vi "Module Top Level.vi"(8 "error in":errorcluster) -> (0 "error out":errorcluster)   [LabVIEW 2020, in "Error Handler.lvlib"]
doc: "This is the top level of the error handler module (a free running module of the ATM simulator). \n\nIt is closed using a user event or a local Stop button. It communicates with the other modules using a\nqueue based API which has comms modules that can be swapped if required."
uses:
  Error Handler.lvlib
  User Events/Controls/UE Abort Action.ctl
  Private Controls/Module Action.ctl
  Private Controls/Module Data Cluster.ctl
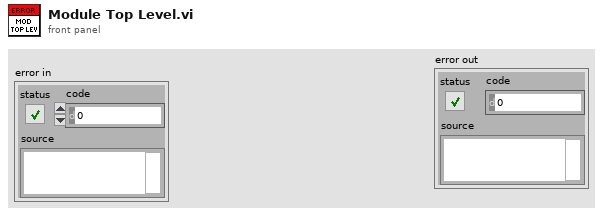
[diagram p1: front panel]
types:
  T1 = typedef "Error Handler.lvlib/Module Data Cluster.ctl" = cluster{"Data":variant, "Action":T2}
  T2 = typedef "Error Handler.lvlib/Module Action.ctl" = enum16{"Process_Step_Err", "Sensor_IO_err", "User_Console_err", "Display_Consol_err", "Error_Log", "Error", "Exit", "Init"}
  T3 = typedef "UE Abort Action.ctl" = enum16{"Destroy", "Get", "Create"}
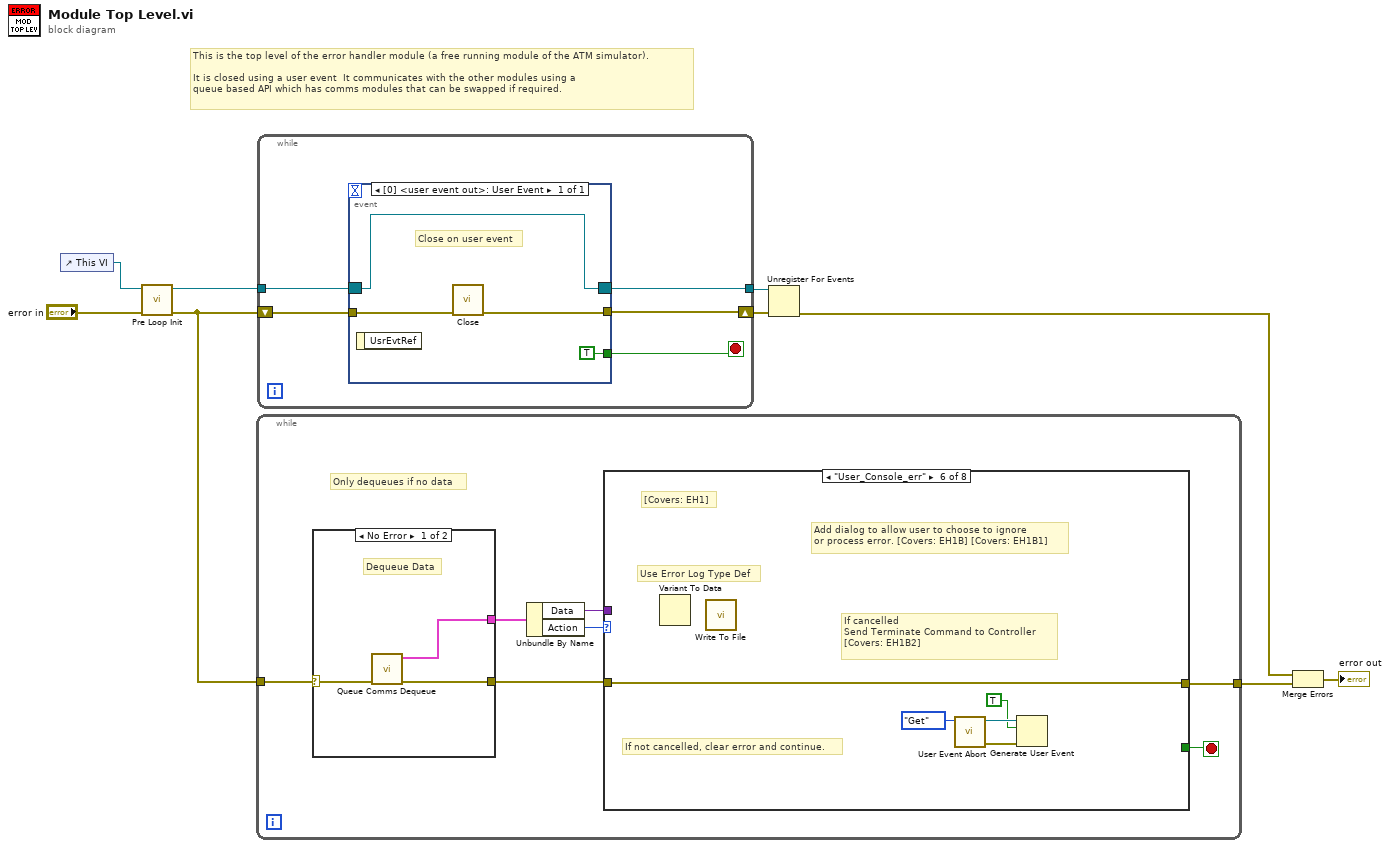
[diagram p0: block diagram]
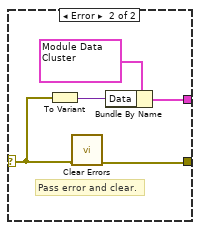
[diagram p2: hidden frame]
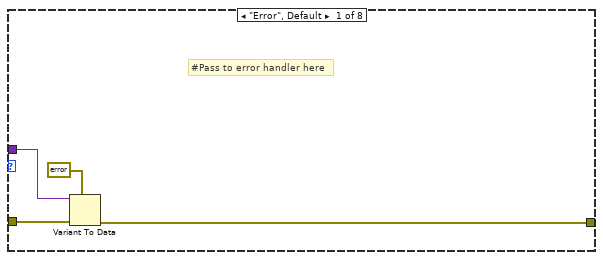
[diagram p3: hidden frame]
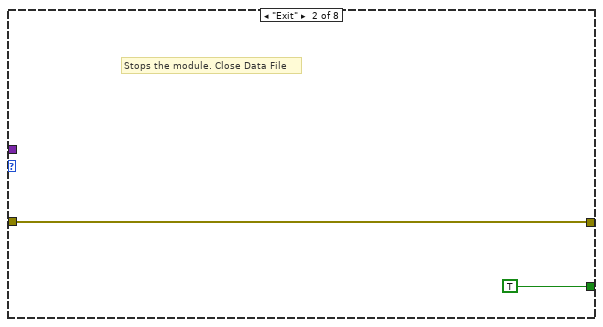
[diagram p4: hidden frame]
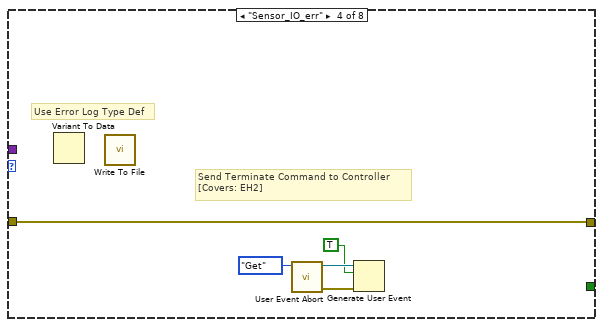
[diagram p6: hidden frame]
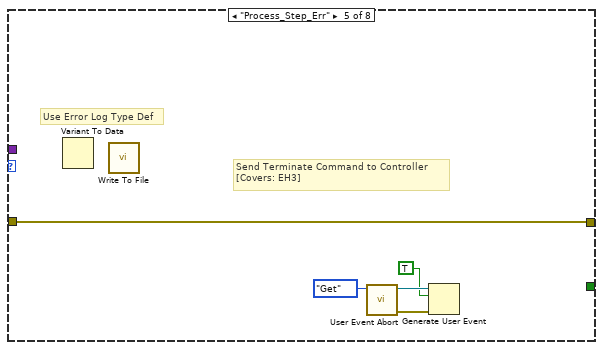
[diagram p7: hidden frame]
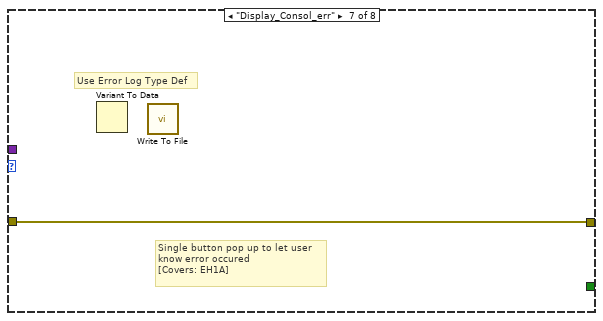
[diagram p8: hidden frame]
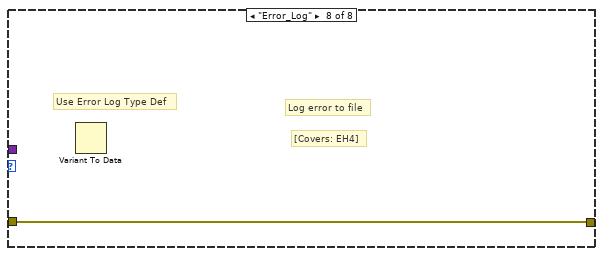
[diagram p9: hidden frame]
diagram:
  # "This is the top level of the error handler module (a free running module of the ATM simulator). \n\nIt is closed using a user event  It communicates with the other modules using a\nqueue based API which has comms modules that can be swapped if required."
  n1 = control-ref of="This VI"() -> (w9:refnum<vi>)
  n2 = call "Pre Loop Init.vi"("error in"="error in", "Ref In"=w9) -> ("error out"=w4:errorcluster, "Event Registration Refnum"=w7:refnum<event-registration>)  [unwired: 8 in]
  n3 = while {
    tunnel: w4 -> [w15]
    tunnel: [w10] -> w2
    stop <- w16 stop-if-true
    # "Only dequeues if no data"
    n4 = case shown="No Error" w15 {
      selector: w15 -> [w18 w21]
      tunnel: [w19 w20] -> w13
      tunnel: [w17 w22] -> w14
      frame No Error {
        # "Dequeue Data"
        n5 = call "Queue Comms Dequeue.vi"("error in"=w18) -> ("error out"=w19:errorcluster, "Data Out"=w17:T1)  [unwired: 9 in]
      }
      frame Error {
        # "Pass error and clear."
        n6 = To Variant(anything=w21) -> (Variant=w23:variant)
        n7 = call <vilib>:"Clear Errors.vi"("error in (no error)"=w21) -> ("error out"=w20:errorcluster)  [unwired: 5 in, 1 out]
        n8 = Bundle By Name(cluster=T1 {"Data"=variant, "Action"=enum."Error"} ("Cluster"), "Data"=w23) -> (w22:T1)
      }
    }
    n9 = Unbundle By Name(w14) -> ("Data"=w11:variant, "Action"=w12:T2)
    n10 = case shown="\"User_Console_err\"" w12 {
      tunnel: [_ TRUE _ _ _ _ _ _] -> w16
      tunnel: w13 -> [w27 w29 w31 w36 w41 w46 w47 w48]
      tunnel: w11 -> [w28 _ _ _ _ _ _ _]
      tunnel: [w26 w29 w31 w36 w41 w46 w47 w48] -> w10
      frame "Error", Default {
        # "#Pass to error handler here"
        n11 = Variant To Data(error in=w27, type=errorcluster {"status"=FALSE, "code"=0, "source"=""} ("error out"), Variant=w28) -> (error out=w26:errorcluster)  [unwired: 1 out]
      }
      frame "Exit" {
        # "Stops the module. Close Data File"
      }
      frame "Init" {
        # "[Covers: EH4]"
        # "Create file, CSV format.  Log description of file, level of error, and \ndate stamp.\nPass File Reference to a shift register"
      }
      frame "Sensor_IO_err" {
        # "Use Error Log Type Def"
        # "Send Terminate Command to Controller\n[Covers: EH2]"
        n12 = Variant To Data() -> ()  [unwired: 3 in, 2 out]
        n13 = call "Write To File.vi"() -> ()  [unwired: 11 in, 1 out]
        n14 = call "User Event Abort.vi"("Action"=UE_Abort_Action."Get") -> ("error out"=w34:errorcluster, "user event out"=w33:refnum<user-event>)  [unwired: 9 in]
        n15 = Generate User Event(user event=w33, event data cluster=TRUE ("event data"), error in=w34) -> ()  [unwired: 1 in, 2 out]
      }
      frame "Process_Step_Err" {
        # "Use Error Log Type Def"
        # "Send Terminate Command to Controller\n[Covers: EH3]"
        n16 = Variant To Data() -> ()  [unwired: 3 in, 2 out]
        n17 = call "Write To File.vi"() -> ()  [unwired: 11 in, 1 out]
        n18 = call "User Event Abort.vi"("Action"=UE_Abort_Action."Get") -> ("error out"=w39:errorcluster, "user event out"=w38:refnum<user-event>)  [unwired: 9 in]
        n19 = Generate User Event(user event=w38, event data cluster=TRUE ("event data"), error in=w39) -> ()  [unwired: 1 in, 2 out]
      }
      frame "User_Console_err" {
        # "[Covers: EH1]"
        # "If not cancelled, clear error and continue."
        # "If cancelled\nSend Terminate Command to Controller\n[Covers: EH1B2]"
        # "Add dialog to allow user to choose to ignore\nor process error. [Covers: EH1B] [Covers: EH1B1]"
        # "Use Error Log Type Def"
        n20 = Variant To Data() -> ()  [unwired: 3 in, 2 out]
        n21 = call "Write To File.vi"() -> ()  [unwired: 11 in, 1 out]
        n22 = call "User Event Abort.vi"("Action"=UE_Abort_Action."Get") -> ("error out"=w44:errorcluster, "user event out"=w43:refnum<user-event>)  [unwired: 9 in]
        n23 = Generate User Event(user event=w43, event data cluster=TRUE ("event data"), error in=w44) -> ()  [unwired: 1 in, 2 out]
      }
      frame "Display_Consol_err" {
        # "Single button pop up to let user\nknow error occured\n[Covers: EH1A]"
        # "Use Error Log Type Def"
        n24 = Variant To Data() -> ()  [unwired: 3 in, 2 out]
        n25 = call "Write To File.vi"() -> ()  [unwired: 11 in, 1 out]
      }
      frame "Error_Log" {
        # "Log error to file"
        # "Use Error Log Type Def"
        # "[Covers: EH4]"
        n26 = Variant To Data() -> ()  [unwired: 3 in, 2 out]
      }
    }
  }
  n27 = while {
    shift-right: [w52] -> w6
    shift-left: w4 -> [w53]
    tunnel: w7 -> [w51]
    tunnel: [w50] -> w5
    stop <- w49 stop-if-true
    n28 = event shown="[0] <user event out>: User Event" {
      selector: w51 -> [w57]
      dyn-events: [w57] -> w50
      timeout: _ -> [_]
      tunnel: w53 -> [w56]
      tunnel: [w55] -> w52
      tunnel: [TRUE ("stop")] -> w49
      event User Event {
        # "Close on user event"
        n29 = event-data() -> ()  [unwired: 1 in, 1 out]
        n30 = call "Close.vi"("error in"=w56) -> ("error out"=w55:errorcluster)  [unwired: 10 in]
      }
    }
  }
  n31 = Unregister For Events(event registration refnum=w5, error in=w6) -> (error out=w1:errorcluster)
  n32 = Merge Errors(w1, w2) -> (→"error out":errorcluster)
